vi "prueba_com_write.vi"() -> ()   [LabVIEW 2021]
uses:
  <vilib>/MakerHub/LINX/Private/Local IO/LinxI2cWrite.vi
  <vilib>/MakerHub/LINX/Public/Utilities/Check Channel.vi
  <vilib>/MakerHub/LINX/Public/Utilities/Open Serial.vi
  <vilib>/MakerHub/LINX/Private/Utilties/Generate Error.vi
  <vilib>/MakerHub/LINX/LMH-LINX.lvlib
panel:
  in  "stop":bool
  out "Device Name 2":string
  out "Error Out 2":errorcluster
  in  "Error In 2":errorcluster
  in  "Serial Port 2":refnum<visa-resource-name>="N/A"
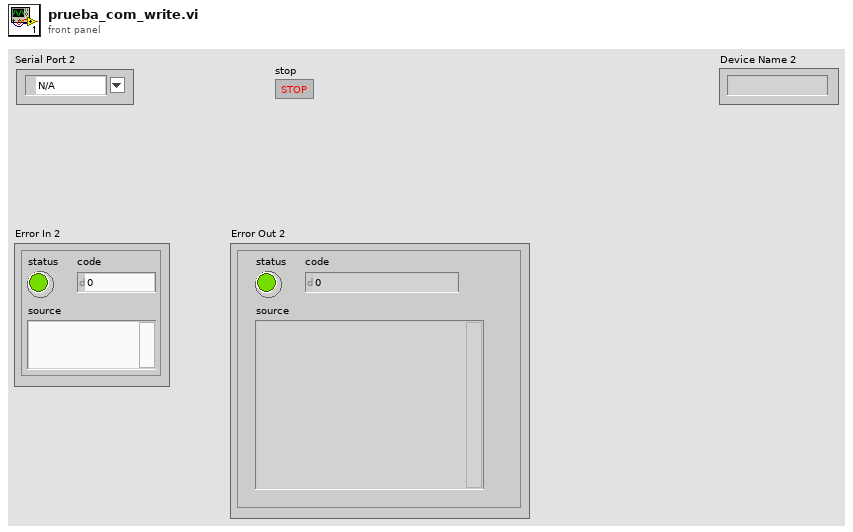
[diagram p1: front panel]
types:
  T1 = typedef "LMH-LINX.lvlib/LINX Ref.ctl" = cluster{"IO":T2, "Interface":T3, "LINX Device Config":T4}
  T2 = typedef "LMH-LINX.lvlib/Platform.ctl" = enum16{"Remote", "Local"}
  T3 = typedef "LMH-LINX.lvlib/Interface.ctl" = enum16{"Serial", "TCP"}
  T4 = typedef "LMH-LINX.lvlib/Device.lvlib/LINX Device Config.ctl" = cluster{"Interface":T3, "COM Port":refnum<visa-resource-name>, "TCP Configuration":T5, "Device Family":u8, "Device ID":u8, "Device Name":string, "TCP Ref":refnum<k5>, "Channels":T6}
  T5 = typedef "LMH-LINX.lvlib/Device.lvlib/TCP Config.ctl" = cluster{"IP Address":string, "Port":u16}
  T6 = typedef "LMH-LINX.lvlib/Channels.ctl" = cluster{"DI":u8[], "DO":u8[], "AI":u8[], "AO":u8[], "PWM":u8[], "QE":u8[], "UART":u8[], "I2C 2":u8[], "SPI":u8[], "CAN":u8[], "Servo":u8[], "AI Ref (V)":dbl, "AI Resolution (Bits)":u8, "AO Ref (V)":dbl, "AO Resolution (Bits)":u8}
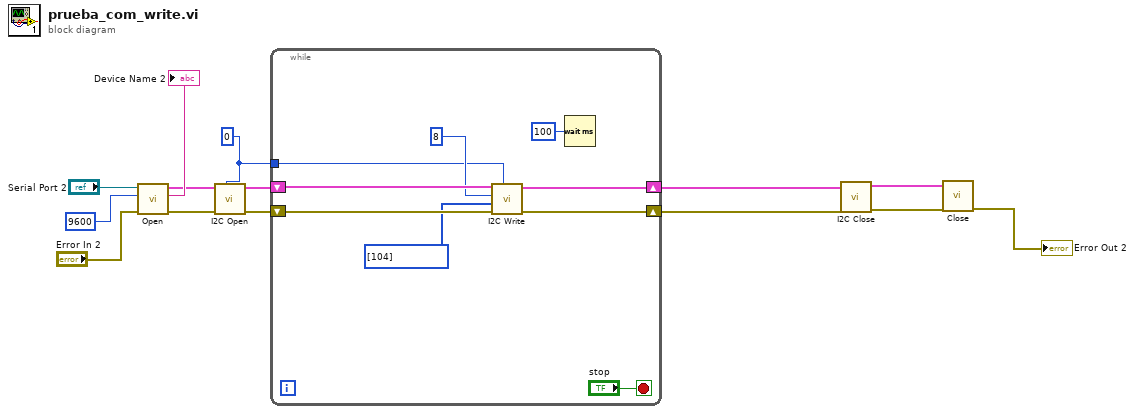
[diagram p0: block diagram]
diagram:
  w4 = u8 0 ("I2C Channel")
  n1 = call-poly <vilib>:"Open.vi"("Error In"="Error In 2", "Baud Rate Override"=u32 9600, "Serial Port"="Serial Port 2") -> ("Error Out"=w9:errorcluster, "Device Name"=→"Device Name 2":string, "LINX Resource"=w3:T1)  [unwired: 6 in]
  n2 = call <vilib>:"I2C Open.vi"("I2C Channel (0)"=w4, "Error In"=w9, "LINX Resource"=w3) -> ("Error Out"=w7:errorcluster, "LINX Resource"=w1:T1)  [unwired: 7 in]
  n3 = while {
    tunnel: w4 -> [w20]
    shift-right: [w17] -> w6
    shift-left: w7 -> [w23]
    shift-right: [w16] -> w5
    shift-left: w1 -> [w22]
    stop <- "stop" stop-if-true
    n4 = call <vilib>:"I2C Write.vi"("I2C Channel"=w20, "Error In"=w23, "Data"=u8[] [104], "I2C Slave Address (0)"=u8 8, "LINX Resource"=w22) -> ("Error Out"=w17:errorcluster, "LINX Resource"=w16:T1)  [unwired: 5 in]
    n5 = Wait (ms)(milliseconds to wait=u32 100) -> ()  [unwired: 1 out]
  }
  n6 = call <vilib>:"I2C Close.vi"("Error In"=w6, "LINX Resource"=w5) -> ("Error Out"=w13:errorcluster, "LINX Resource"=w12:T1)  [unwired: 8 in]
  n7 = call <vilib>:"Close.vi"("Error In"=w13, "LINX Resource"=w12) -> ("Error Out"=→"Error Out 2":errorcluster)  [unwired: 9 in]
